vi "Setting Up.vi"(4 "Async Elements":refnum<class "Async Elements.lvclass">, 6 "This VI":refnum<vi>, 7 "Actor in":refnum<class "Actor.lvclass">, 10 "Refs":refnum<class "Refs.lvclass">) -> (0 "Error out":errorcluster, 2 "Msg Ref":refnum<event-registration>, 5 "Actor out":refnum<class "Actor.lvclass">)   [LabVIEW 2020, in "jettl.lvlib" / "Event Transport.lvlib"]
uses:
  Event Transport.lvlib
  Actor/Actor.lvclass
  Refs/Refs.lvclass
  Msg/Msg.lvclass
  Async Elements/Async Elements.lvclass
  Event Transport/Event Transport.lvclass
  jettl.lvlib
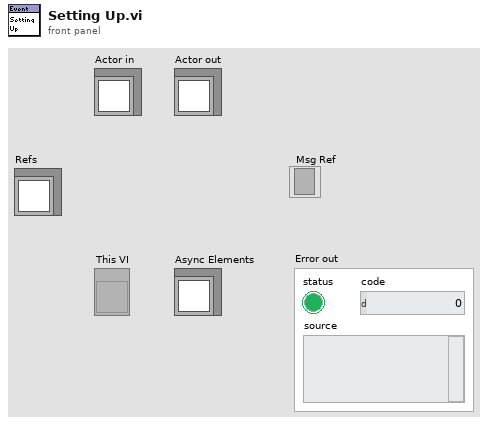
[diagram p1: front panel]
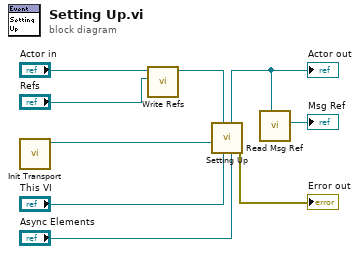
[diagram p0: block diagram]
diagram:
  n1 = call "Init Transport.vi"() -> ("Event Transport out"=w1:refnum<class "Event Transport.lvclass">)  [unwired: 11 in]
  n2 = call-dynamic "Write Refs.vi"("Refs"="Refs", "Actor in"="Actor in") -> ("Actor out"=w7:refnum<class "Actor.lvclass">)  [unwired: 9 in]
  n3 = call "Setting Up.vi"("Async Elements"="Async Elements", "This VI"="This VI", "Actor in"=w7, "Transport"=w1) -> ("Error out"=→"Error out":errorcluster, "Actor out"=w5:refnum<class "Actor.lvclass">)  [unwired: 6 in]
  "Actor out" <- w5
  n4 = call "Read Msg Ref.vi"("Actor"=w5) -> ("Msg Ref"=→"Msg Ref":refnum<event-registration>)  [unwired: 10 in]
